vi "counter_quad_w_index.vi"(4 "Enable Index":bool, 6 "Reset":bool, 7 "A":bool, 10 "Z":bool, 11 "B":bool) -> (3 "Position (counts)":i32)   [LabVIEW 2011]
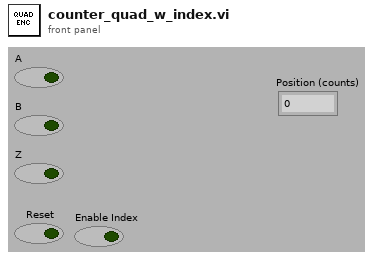
[diagram p1: front panel]
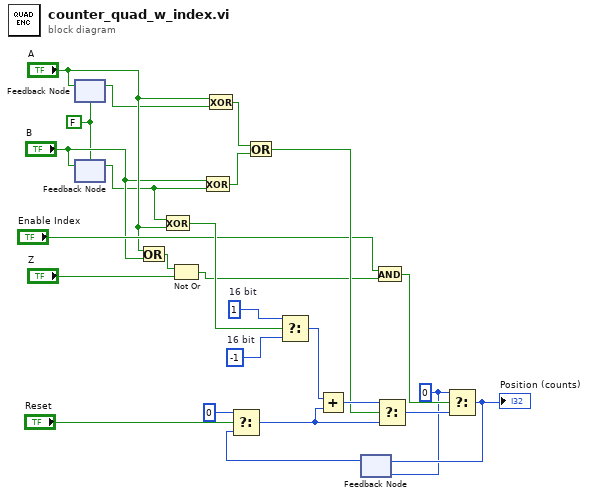
[diagram p0: block diagram]
diagram:
  w4 = FALSE
  w1 = 0 ("t")
  w19 = -1  # 16 bit
  w20 = 1  # 16 bit
  n1 = feedback-in #1("A") -> ()
  n2 = feedback #1(w4) -> (w7:bool)
  n3 = feedback #2(w4) -> (w5:bool)
  n4 = feedback-in #2("B") -> ()
  n5 = Or(x="A", y="B") -> (x .or. y?=w15:bool)
  n6 = Exclusive Or(1:"A", 2:w5) -> (0:w13:bool)
  n7 = Not Or(1:"Z", 2:w15) -> (0:w12:bool)
  n8 = Exclusive Or(1:w5, 2:"B") -> (0:w17:bool)
  n9 = Exclusive Or(1:w7, 2:"A") -> (0:w16:bool)
  n10 = Or(x=w16, y=w17) -> (x .or. y?=w14:bool)
  n11 = Select(t=w20, s=w13, f=w19) -> (s? t:f=w21:i32)
  n12 = feedback #3(w1) -> (w3:i32)
  n13 = Select(t=0, s="Reset", f=w3) -> (s? t:f=w23:i32)
  n14 = Add(x=w21, y=w23) -> (x+y=w24:i32)
  n15 = And(x="Enable Index", y=w12) -> (x .and. y?=w10:bool)
  n16 = Select(t=w24, s=w14, f=w23) -> (s? t:f=w18:i32)
  n17 = Select(t=w1, s=w10, f=w18) -> (s? t:f=w2:i32)
  "Position (counts)" <- w2
  n18 = feedback-in #3(w2) -> ()
